vi "Load and Play Path.vi"(6 "filename":string, 7 "Command Info In":T1, 8 "Is Blue Alliance? in":bool=TRUE, 9 "Set IMU?":bool, 10 "Path":path) -> (0 "Command Info Out":T1)   [LabVIEW 2023]
uses:
  <vilib>/Rock Robotics/WPI/Framework/Command Status Info.ctl
  <vilib>/Rock Robotics/WPI/Framework/Completion Status.ctl
  <vilib>/Rock Robotics/WPI/Framework/Completion Notifier.ctl
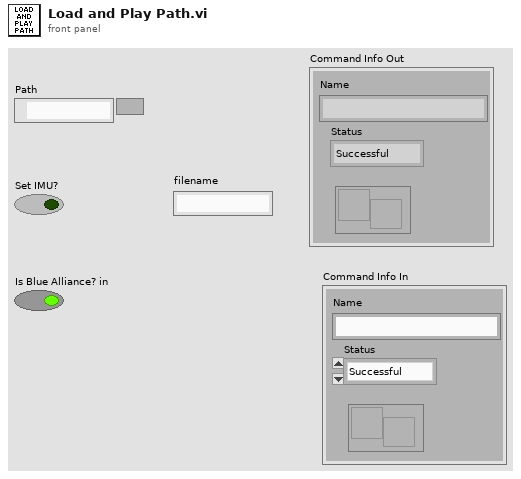
[diagram p1: front panel]
types:
  T1 = typedef "Command Status Info.ctl" = cluster{"Name":string, "Status":T2, "notifier out":T3}
  T2 = typedef "Completion Status.ctl" = enum16{"Successful", "Aborted", "Incomplete"}
  T3 = typedef "Completion Notifier.ctl" = refnum<notifier>
  T4 = cluster{dbl, "Command out":cluster{"Name":string, "vi reference":refnum<vi>, i32[], variant[]}}[]
  T5 = typedef "Robot Velocities.ctl" = cluster{"X Velocity":dbl, "Y Velocity":dbl, "Rotational \nVelocity":dbl}
  T6 = typedef "CTRE_PigeonIMU_DeviceRef.ctl" = cluster{"DeviceStatus":errorcluster, "Device Number":u8, "Type":T7, "Device ID":u32, "Handle":u64, "UsageFrame":u32, "Library Path":path}
  T7 = typedef "CTRE_PigeonIMU_ConnectionType.ctl" = u32
  T8 = cluster{"Velocities":T5[], "Positions":cluster{"x":dbl, "y":dbl, "th":dbl}[], cluster{dbl, "Command out":cluster{"Name":string, "vi reference":refnum<vi>, i32[], variant[]}}[], "Zero Velocity?":bool[]}
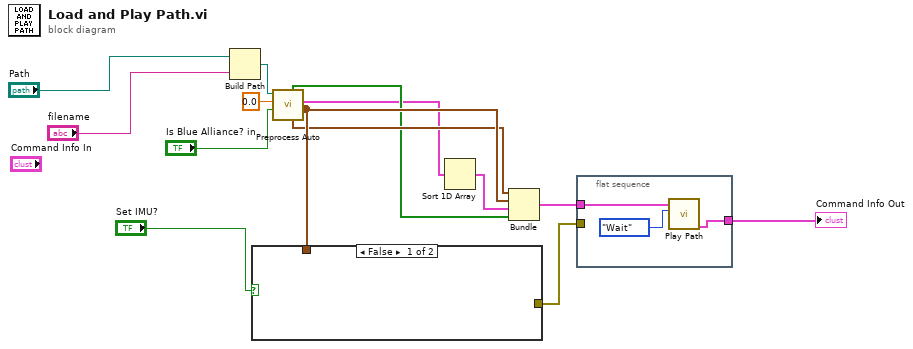
[diagram p0: block diagram]
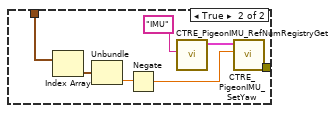
[diagram p2: hidden frame]
diagram:
  n1 = Build Path(base path="Path", name or relative path="filename") -> (appended path=w13:path)
  n2 = call "Preprocess Auto.vi"("Is Blue Alliance?"="Is Blue Alliance? in", "Start Time"=0.0, "appended path"=w13) -> ("Positions"=w8:cluster{"x":dbl, "y":dbl, "th":dbl}[], "Array"=w4:T4, "Velocities"=w7:T5[], "Zero Velocity?"=w6:bool[])  [unwired: 4 in, 1 out]
  n3 = case shown="False" "Set IMU?" {
    tunnel: w8 -> [_ w16]
    tunnel: [_ w15] -> w11
    frame False {
    }
    frame True {
      n4 = Index Array(array=w16) -> (element=w19:cluster{"x":dbl, "y":dbl, "th":dbl})  [unwired: 1 in]
      n5 = Unbundle(w19) -> ("th"=w18:dbl)  [unwired: 2 out]
      n6 = Negate(x=w18) -> (-x=w17:dbl)
      n7 = call <vilib>:"CTRE_PigeonIMU_RefNumRegistryGet.vi"("refnum name"="IMU") -> ("PigeonIMUDevRef"=w21:T6)  [unwired: 9 in, 1 out]
      n8 = call <vilib>:"CTRE_PigeonIMU_SetYaw.vi"("Value"=w17, "PigeonIMUDevRef"=w21) -> ("error out"=w15:errorcluster)  [unwired: 8 in, 1 out]
    }
  }
  n9 = Sort 1D Array(array=w4) -> (sorted array=w5:T4)
  n10 = Bundle("Velocities"=w7, "Positions"=w8, w5, "Zero Velocity?"=w6) -> (w10:T8)  [unwired: 1 in]
  n11 = flat-sequence {
    tunnel: w10 -> [w23]
    tunnel: w11 -> [_]
    tunnel: [w22] -> w2
    frame #0 {
      n12 = call "Play Path.vi"("Synchronization"=enum16{"Start", "Wait"}."Wait", "Auto Data"=w23) -> ("Command Info Out"=w22:T1)  [unwired: 9 in]
    }
  }
  "Command Info Out" <- w2
